vi "test Add Find Remove EST CD.vi"(8 "error in (no error)":errorcluster, 11 "TestCase in":refnum<class "Scripting API Test Case.lvclass">) -> (0 "error out":errorcluster, 3 "TestCase out":refnum<class "Scripting API Test Case.lvclass">)   [LabVIEW 2017, in "Scripting API Test Case.lvclass"]
uses:
  Scripting API Test Case.lvclass
  Scripting API/Custom Device/Engine Simulation Toolkit Custom Device Settings.ctl
  Scripting API Test Case.lvclass/Scripting API Test Case.ctl
  <vilib>/addons/_JKI Toolkits/VI Tester/TestCase.llb/TestCase.lvclass
  Scripting API/Engine Simulation Toolkit Scripting API.lvlib
  C:/Program Files (x86)/National Instruments/LabVIEW 2017/vi.lib/addons/_JKI Toolkits/VI Tester/TestCase.llb/TestCase.lvclass
panel:
  in  "Save?":bool
  out "Output Filename":string
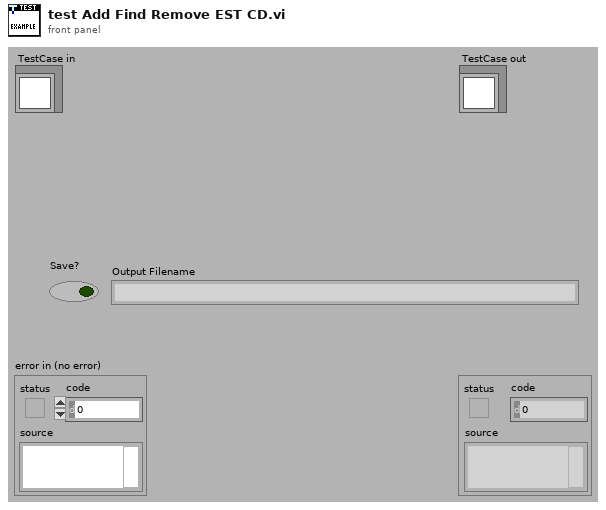
[diagram p1: front panel]
types:
  T1 = typedef "Engine Simulation Toolkit Scripting API.lvlib/Engine Simulation Toolkit Custom Device Settings.ctl" = cluster{"Name":string, "Execution priority":enum16{"Low", "Medium", "High"}, "Rate decimation":i32, "CPU":i32}
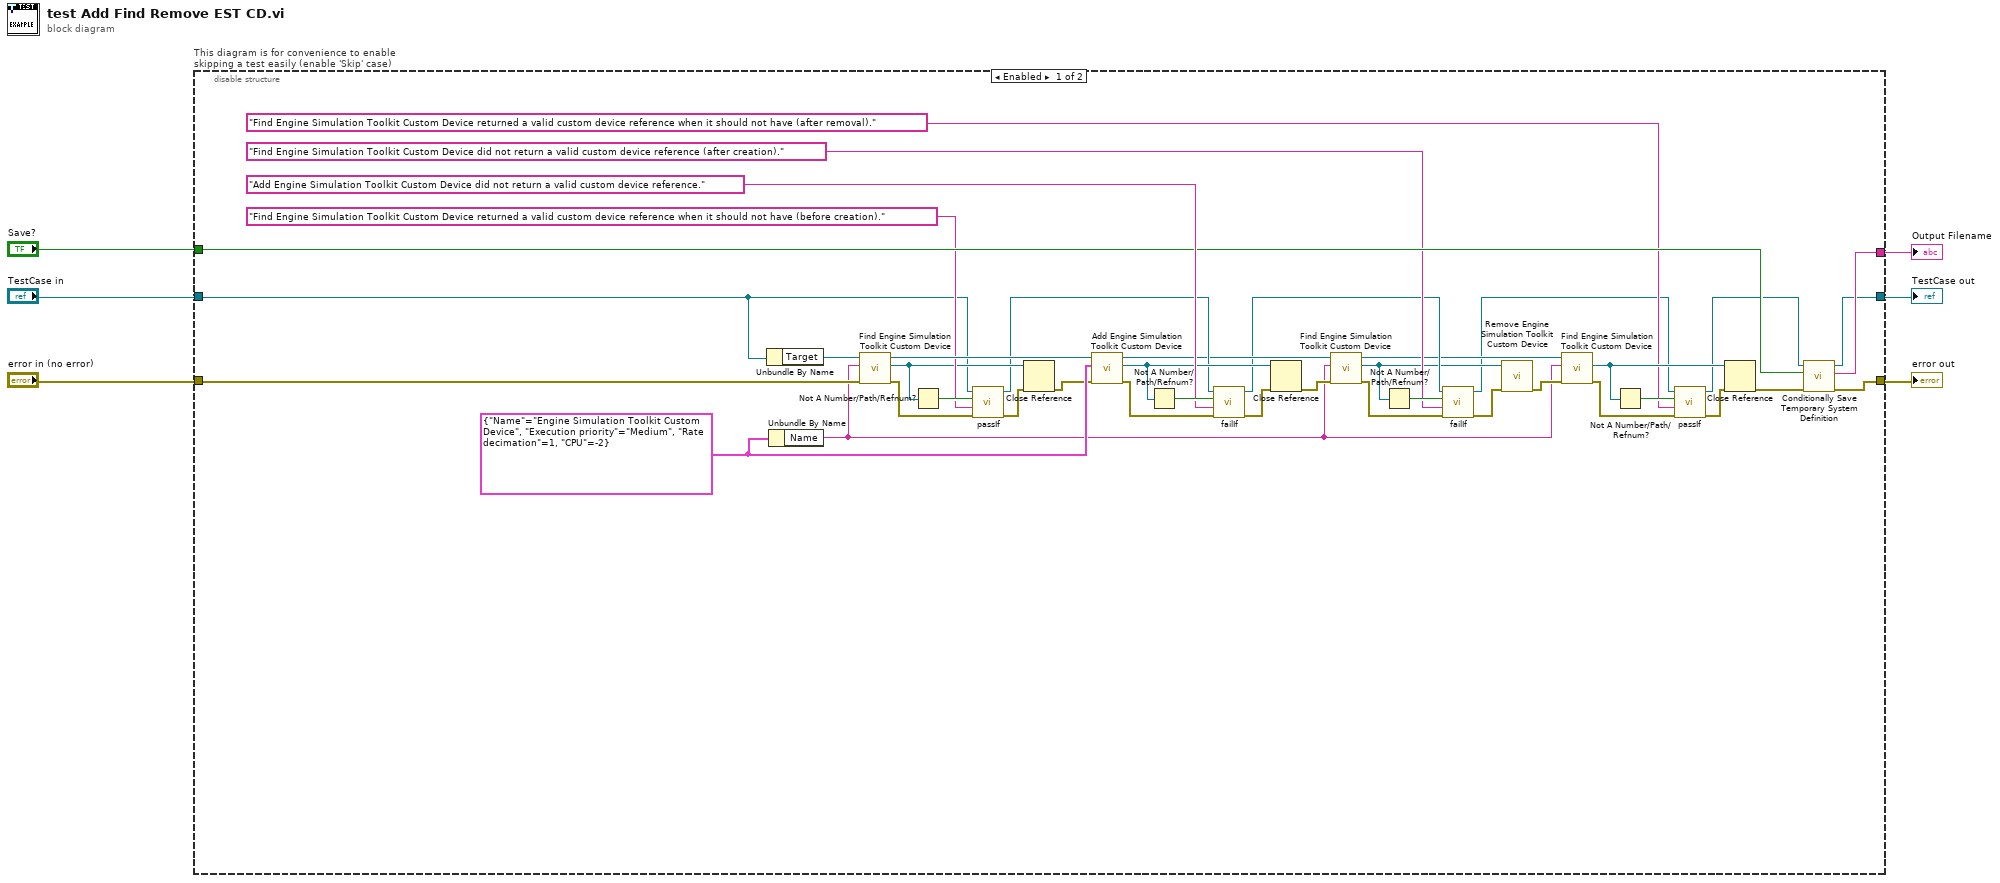
[diagram p0: block diagram]
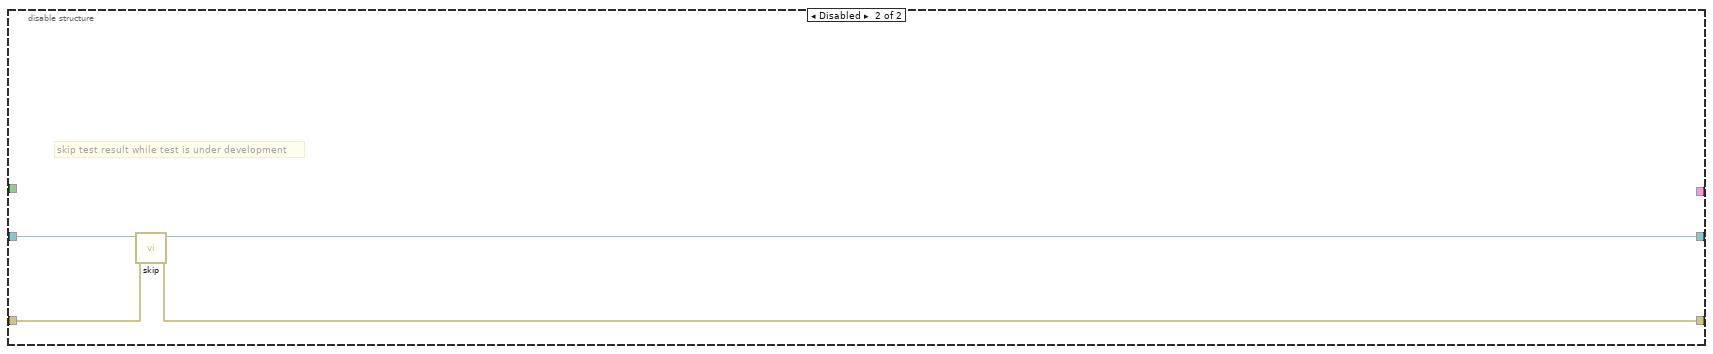
[diagram p2: hidden frame]
diagram:
  n1 = disable-structure "This diagram is for convenience to enable skipping a test easily (enable 'Skip' case)" shown="Enabled" {
    disable-tunnel: "TestCase in" -> [w11 w50]
    disable-tunnel: [w7 w48] -> w3
    disable-tunnel: [w9 w49] -> w5
    disable-tunnel: "error in (no error)" -> [w46 w47]
    disable-tunnel: [w40 _] -> w2
    disable-tunnel: "Save?" -> [w39 _]
    frame Enabled {
      w37 = T1 {"Name"="Engine Simulation Toolkit Custom Device", "Execution priority"=enum."Medium", "Rate decimation"=1, "CPU"=-2} ("Engine Simulation Toolkit Custom Device Settings")
      n2 = Unbundle By Name(w11) -> ("Target"=w10:refnum<k24>)
      n3 = Unbundle By Name(w37) -> ("Name"=w12:string)
      n4 = call "Find Engine Simulation Toolkit Custom Device.vi"("error in (no error)"=w46, "Name"=w12, "Target in"=w10) -> ("error out"=w35:errorcluster, "EST Custom Device"=w33:refnum<k24>, "Target out"=w38:refnum<k24>)  [unwired: 6 in]
      n5 = Not A Number/Path/Refnum?(number/path/refnum=w33) -> (NaN/Path/Refnum?=w36:bool)
      n6 = call-dynamic "passIf.vi"("error in (no error)"=w35, "message (\"\")"="Find Engine Simulation Toolkit Custom Device returned a valid custom device reference when it should not have (before creation)." ("message (\"\")"), "pass"=w36, "TestCase in"=w11) -> ("error out"=w32:errorcluster, "TestCase out"=w30:refnum<class "Scripting API Test Case.lvclass">)  [unwired: 6 in]
      n7 = Close Reference(reference=w33, error in (no error)=w32) -> (error out=w31:errorcluster)
      n8 = call "Add Engine Simulation Toolkit Custom Device.vi"("error in (no error)"=w31, "Settings"=w37, "Target in"=w38) -> ("error out"=w44:errorcluster, "EST Custom Device"=w42:refnum<k24>, "Target out"=w26:refnum<k24>)  [unwired: 6 in]
      n9 = Not A Number/Path/Refnum?(number/path/refnum=w42) -> (NaN/Path/Refnum?=w45:bool)
      n10 = call-dynamic "failIf.vi"("error in (no error)"=w44, "message (\"\")"="Add Engine Simulation Toolkit Custom Device did not return a valid custom device reference." ("message (\"\")"), "fail"=w45, "TestCase in"=w30) -> ("error out"=w41:errorcluster, "TestCase out"=w24:refnum<class "Scripting API Test Case.lvclass">)  [unwired: 6 in]
      n11 = Close Reference(reference=w42, error in (no error)=w41) -> (error out=w27:errorcluster)
      n12 = call "Find Engine Simulation Toolkit Custom Device.vi"("error in (no error)"=w27, "Name"=w12, "Target in"=w26) -> ("error out"=w28:errorcluster, "EST Custom Device"=w23:refnum<k24>, "Target out"=w17:refnum<k24>)  [unwired: 6 in]
      n13 = Not A Number/Path/Refnum?(number/path/refnum=w23) -> (NaN/Path/Refnum?=w29:bool)
      n14 = call-dynamic "failIf.vi"("error in (no error)"=w28, "message (\"\")"="Find Engine Simulation Toolkit Custom Device did not return a valid custom device reference (after creation)." ("message (\"\")"), "fail"=w29, "TestCase in"=w24) -> ("error out"=w22:errorcluster, "TestCase out"=w13:refnum<class "Scripting API Test Case.lvclass">)  [unwired: 6 in]
      n15 = call "Remove Engine Simulation Toolkit Custom Device.vi"("error in (no error)"=w22, "EST Custom Device"=w23) -> ("error out"=w16:errorcluster)  [unwired: 9 in]
      n16 = call "Find Engine Simulation Toolkit Custom Device.vi"("error in (no error)"=w16, "Name"=w12, "Target in"=w17) -> ("error out"=w20:errorcluster, "EST Custom Device"=w19:refnum<k24>)  [unwired: 6 in, 1 out]
      n17 = Not A Number/Path/Refnum?(number/path/refnum=w19) -> (NaN/Path/Refnum?=w21:bool)
      n18 = call-dynamic "passIf.vi"("error in (no error)"=w20, "message (\"\")"="Find Engine Simulation Toolkit Custom Device returned a valid custom device reference when it should not have (after removal)." ("message (\"\")"), "pass"=w21, "TestCase in"=w13) -> ("error out"=w18:errorcluster, "TestCase out"=w8:refnum<class "Scripting API Test Case.lvclass">)  [unwired: 6 in]
      n19 = Close Reference(reference=w19, error in (no error)=w18) -> (error out=w15:errorcluster)
      n20 = call "Conditionally Save Temporary System Definition.vi"("error in (no error)"=w15, "Save?"=w39, "Test Case"=w8) -> ("error out"=w9:errorcluster, "filename"=w40:string, "Test Case"=w7:refnum<class "Scripting API Test Case.lvclass">)  [unwired: 6 in]
    }
    frame Disabled {
      # "skip test result while test is under development"
      n21 = call <vilib>:"skip.vi"("error in (no error)"=w47, "TestCase in"=w50) -> ("error out"=w49:errorcluster, "TestCase out"=w48:refnum<class "Scripting API Test Case.lvclass">)  [unwired: 8 in]
    }
  }
  "error out" <- w5
  "TestCase out" <- w3
  "Output Filename" <- w2
